vi "Configure Trigger (Setup and Hold Time).vi"(0 "VISA resource name":refnum<visa-resource-name>, 1 "Hold Time (1E-9 s)":dbl=1e-09, 2 "Setup Time (1E-9 s)":dbl=1e-09, 5 "Trigger Source (1: Channel1)":i32(ring)=1 items=["Channel1"=1, "Channel2"=2, "Channel3"=3, "Channel4"=4], 7 "Data Source (2: Channel2)":i32(ring)=2 items=["Channel1"=1, "Channel2"=2, "Channel3"=3, "Channel4"=4], 9 "Clock Source Trigger Edge (0: Rising)":i32(ring) items=["Rising", "Falling"], 11 "error in (no error)":errorcluster, 12 "Violation Mode (0: Setup Time)":i32(ring) items=["Setup Time", "Hold Time", "Setup and Hold Time"]) -> (4 "VISA resource name out":refnum<visa-resource-name>, 15 "error out":errorcluster)   [LabVIEW 2020, in "Agilent 90000 Series.lvlib"]
doc: "Configures the setup and hold time violation trigger parameters."
uses:
  Agilent 90000 Series.lvlib
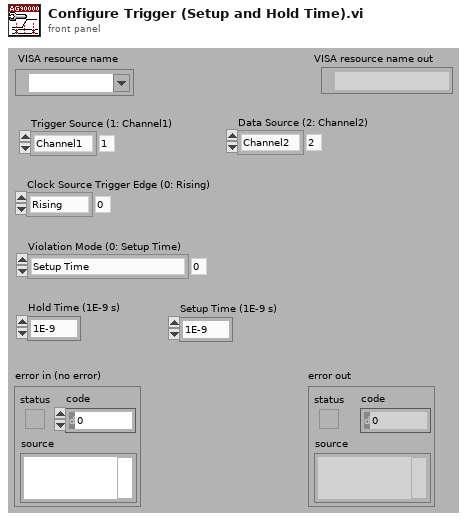
[diagram p1: front panel]
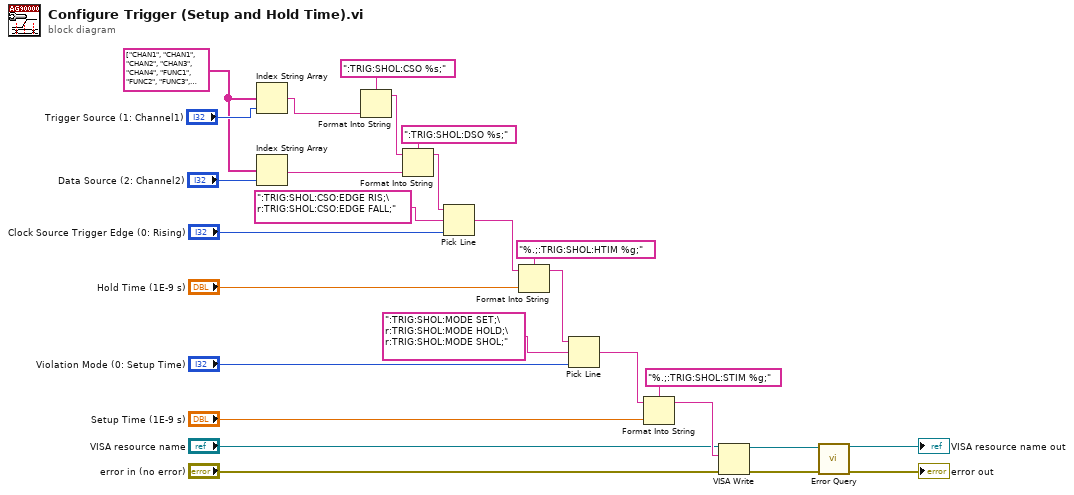
[diagram p0: block diagram]
diagram:
  w5 = string[] ["CHAN1", "CHAN1", "CHAN2", "CHAN3", "CHAN4", "FUNC1", "FUNC2", "FUNC3", "FUNC4", "WMEM1", "WMEM2", "WMEM3", "WMEM4", "AUX", "LINE"]
  n1 = Index String Array(1:"Trigger Source (1: Channel1)", 2:w5) -> (0:w7:string)  [unwired: 1 out]
  n2 = Index String Array(1:"Data Source (2: Channel2)", 2:w5) -> (0:w1:string)  [unwired: 1 out]
  n3 = Format Into String(format string=":TRIG:SHOL:CSO %s;", w7) -> (resulting string=w6:string)  [unwired: 2 in, 1 out]
  n4 = Format Into String(format string=":TRIG:SHOL:DSO %s;", initial string=w6, w1) -> (resulting string=w3:string)  [unwired: 1 in, 1 out]
  n5 = Pick Line(string ("")=w3, multi-line string=":TRIG:SHOL:CSO:EDGE RIS;\r:TRIG:SHOL:CSO:EDGE FALL;", line index="Clock Source Trigger Edge (0: Rising)") -> (output string=w25:string)
  n6 = Format Into String(format string="%.;:TRIG:SHOL:HTIM %g;", initial string=w25, "Hold Time (1E-9 s)") -> (resulting string=w22:string)  [unwired: 1 in, 1 out]
  n7 = Pick Line(string ("")=w22, multi-line string=":TRIG:SHOL:MODE SET;\r:TRIG:SHOL:MODE HOLD;\r:TRIG:SHOL:MODE SHOL;", line index="Violation Mode (0: Setup Time)") -> (output string=w19:string)
  n8 = Format Into String(format string="%.;:TRIG:SHOL:STIM %g;", initial string=w19, "Setup Time (1E-9 s)") -> (resulting string=w16:string)  [unwired: 1 in, 1 out]
  n9 = VISA Write(VISA resource name="VISA resource name", write buffer=w16, error in (no error)="error in (no error)") -> (VISA resource name out=w13:refnum<visa-resource-name>, error out=w12:errorcluster)  [unwired: 1 out]
  n10 = call "Error Query.vi"("error in (no error)"=w12, "VISA resource name"=w13) -> ("error out"=→"error out":errorcluster, "VISA resource name out"=→"VISA resource name out":refnum<visa-resource-name>)  [unwired: 8 out]
